vi "Set_Adam_Watchdogs.vi"(1 "Set Watchdogs":bool) -> (0 "Error String":string)   [LabVIEW 2016]
uses:
  Anemometry/Anemometry Sub Vis/Globals/Constants_global.vi
panel:
  out "Day Time":bool
  out "Display":string[][](table)
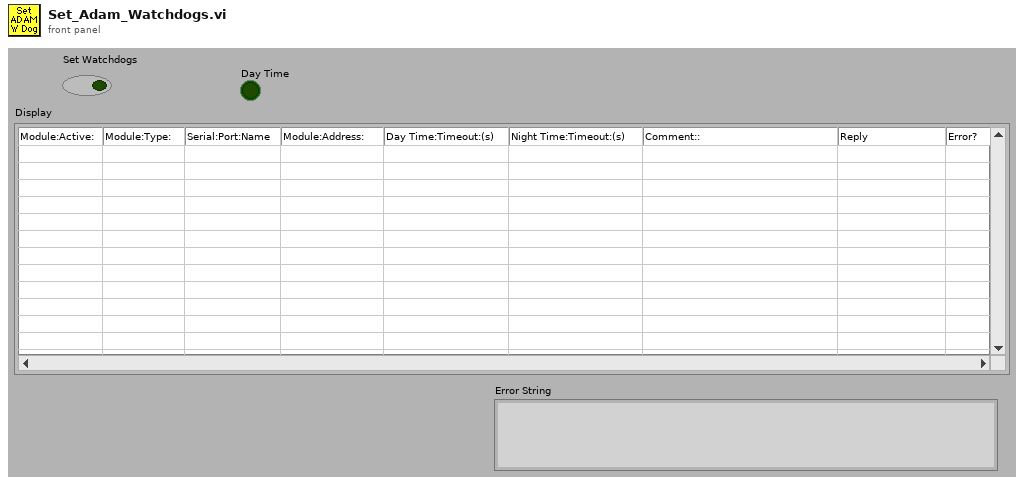
[diagram p1: front panel]
types:
  T1 = typedef "LVDateTimeRec.ctl" = cluster{"fractional second":dbl, "second":i32, "minute":i32, "hour":i32, "day of month":i32, "month":i32, "year":i32, "day of week":i32, "day of year":i32, "DST":i32}
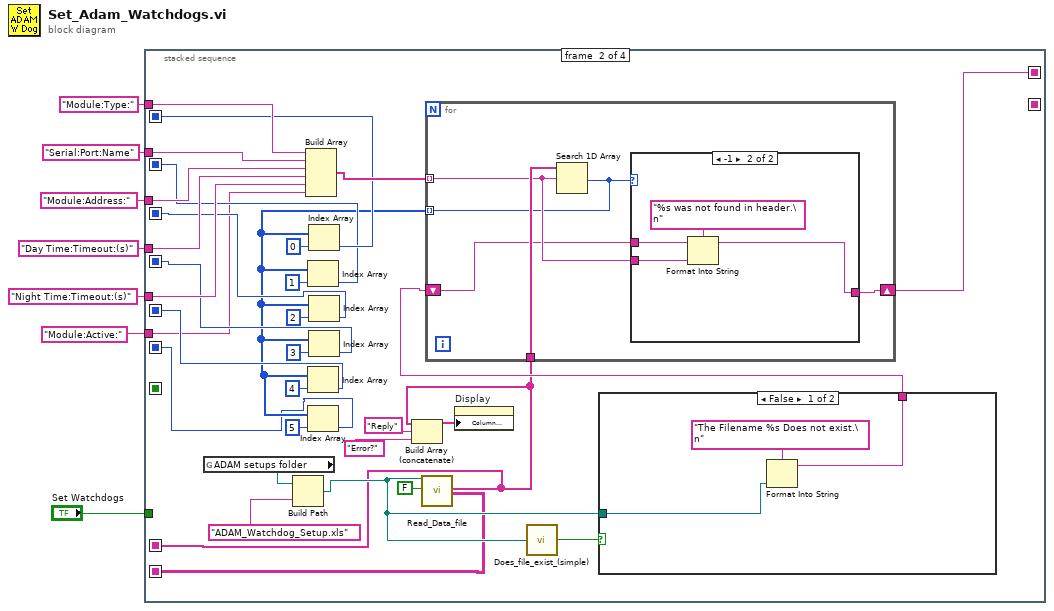
[diagram p0: block diagram]
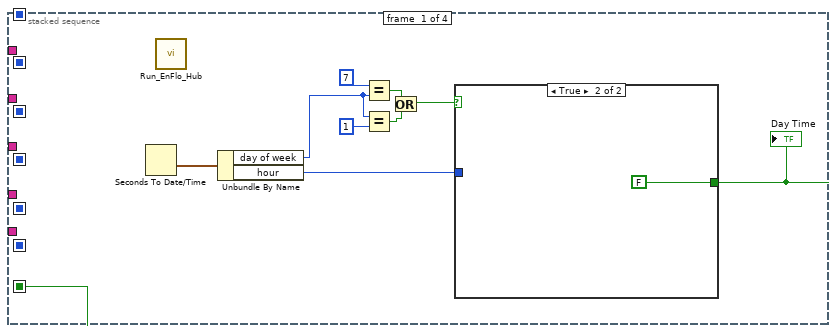
[diagram p2: hidden frame]
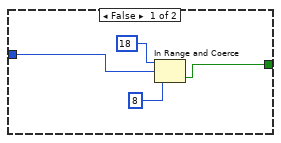
[diagram p3: hidden frame]
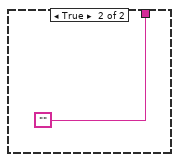
[diagram p4: hidden frame]
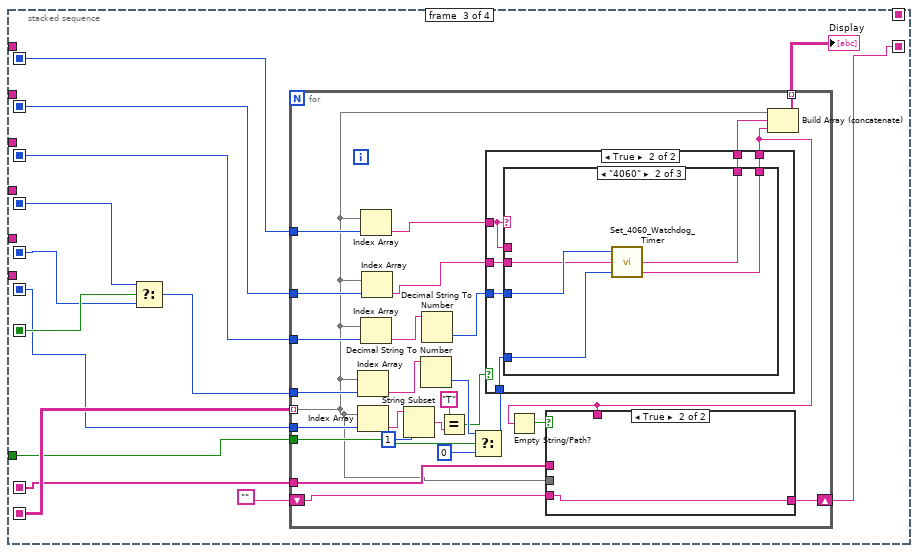
[diagram p6: hidden frame]
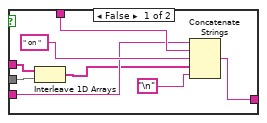
[diagram p7: hidden frame]
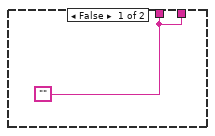
[diagram p8: hidden frame]
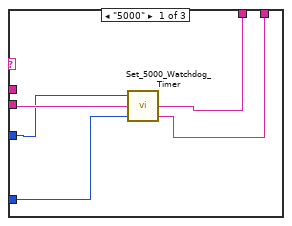
[diagram p9: hidden frame]
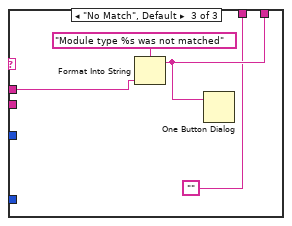
[diagram p10: hidden frame]
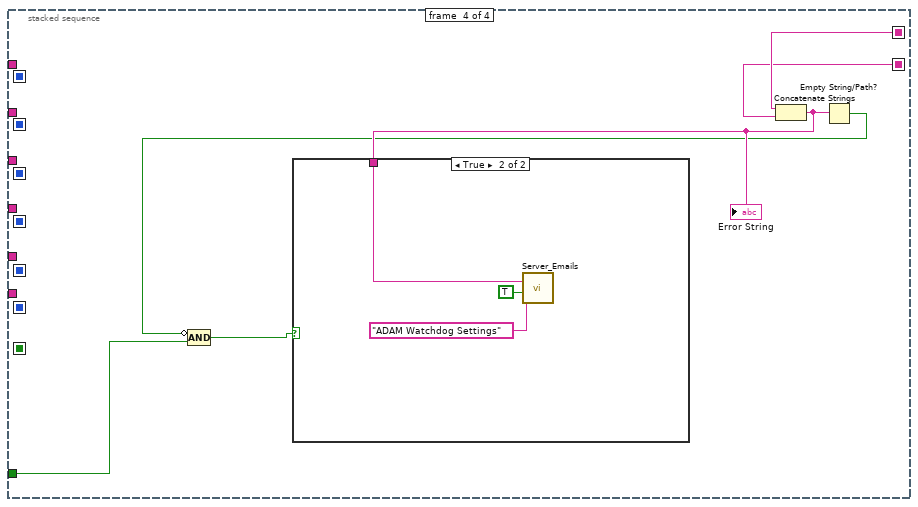
[diagram p11: hidden frame]
diagram:
  n1 = stacked-sequence {
    seq-local: [w8 _ _ _] -> [_ _ w80 _]
    seq-local: [_ w36 _ _] -> [_ _ w78 _]
    seq-local: [_ w35 _ _] -> [_ _ w77 _]
    seq-local: [_ w34 _ _] -> [_ _ w76 _]
    seq-local: [_ w33 _ _] -> [_ _ w75 _]
    seq-local: [_ w32 _ _] -> [_ _ w74 _]
    seq-local: [_ w42 _ _] -> [_ _ _ w144]
    seq-local: [_ w31 _ _] -> [_ _ w79 _]
    seq-local: [_ _ w71 _] -> [_ _ _ w143]
    seq-local: [_ w24 _ _] -> [_ _ w69 _]
    seq-local: [_ w23 _ _] -> [_ _ w68 _]
    tunnel: "Module:Type:" -> [_ w51 _ _]
    tunnel: "Serial:Port:Name" -> [_ w50 _ _]
    tunnel: "Module:Address:" -> [_ w49 _ _]
    tunnel: "Day Time:Timeout:(s)" -> [_ w48 _ _]
    tunnel: "Night Time:Timeout:(s)" -> [_ w47 _ _]
    tunnel: "Set Watchdogs" -> [_ _ w70 w141]
    tunnel: "Module:Active:" -> [_ w27 _ _]
    frame #0 {
      n2 = Seconds To Date/Time() -> (date time rec=w9:T1)  [unwired: 2 in]
      n3 = call "Run_EnFlo_Hub.vi"() -> ()  [unwired: 7 in, 1 out]
      n4 = Unbundle By Name(w9) -> ("day of week"=w11:i32, "hour"=w16:i32)
      n5 = Equal?(x=7, y=w11) -> (x = y?=w13:bool)
      n6 = Equal?(x=w11, y=1) -> (x = y?=w14:bool)
      n7 = Or(x=w13, y=w14) -> (x .or. y?=w15:bool)
      n8 = case shown="True" w15 {
        tunnel: w16 -> [w20 _]
        tunnel: [w17 FALSE] -> w8
        frame False {
          n9 = In Range and Coerce(upper limit=18, x=w20, lower limit=8) -> (In Range?=w17:bool)  [unwired: 1 out]
        }
        frame True {
        }
      }
      "Day Time" <- w8
    }
    frame #1 {
      n10 = global read "Constants_global.vi" "ADAM setups folder"() -> (w53:path)
      n11 = Build Path(base path=w53, name or relative path="ADAM_Watchdog_Setup.xls") -> (appended path=w44:path)
      n12 = Build Array(w51, w50, w49, w48, w47, w27) -> (w46:string[])
      n13 = call "Read_Data_file.vi"("Results file"=w44, "Delete First Rows?"=FALSE) -> ("Ch names Out"=w23:string[], "Channel Values Out"=w31:string[][])  [unwired: 7 in, 9 out]
      n14 = Build Array (concatenate)(w23, "Reply", "Error?" ("element")) -> (w29:string[])
      n15 = property on="Display" class="Tbl (strict)"("Column Headers[]"=w29) -> ()  [unwired: 2 in, 2 out]
      n16 = call "Does_file_exist_(simple).vi"("Pathname"=w44) -> ("exists?"=w45:bool)
      n17 = case shown="False" w45 {
        tunnel: w44 -> [w56 _]
        tunnel: [w54 ""] -> w43
        frame False {
          n18 = Format Into String(format string="The Filename %s Does not exist.\n", w56) -> (resulting string=w54:string)  [unwired: 2 in, 1 out]
        }
        frame True {
        }
      }
      n19 = for {
        tunnel: w23 -> [w62]
        tunnel: w46 -> [w61] mode=indexing
        shift-right: [w59] -> w42
        shift-left: w43 -> [w60]
        tunnel: [w58] -> w25 mode=indexing
        n20 = Search 1D Array(1D array=w62, element=w61) -> (index of element=w58:i32)  [unwired: 1 in]
        n21 = case shown="-1" w58 {
          tunnel: w61 -> [_ w67]
          tunnel: w60 -> [w63 w65]
          tunnel: [w63 w64] -> w59
          frame 0, Default {
          }
          frame -1 {
            n22 = Format Into String(format string="%s was not found in header.\n", initial string=w65, w67) -> (resulting string=w64:string)  [unwired: 1 in, 1 out]
          }
        }
      }
      n23 = Index Array(array=w25, index=1) -> (element=w35:i32)
      n24 = Index Array(array=w25, index=4) -> (element=w32:i32)
      n25 = Index Array(array=w25, index=5) -> (element=w24:i32)
      n26 = Index Array(array=w25, index=0) -> (element=w36:i32)
      n27 = Index Array(array=w25, index=2) -> (element=w34:i32)
      n28 = Index Array(array=w25, index=3) -> (element=w33:i32)
    }
    frame #2 {
      n29 = Select(t=w75, s=w80, f=w74) -> (s? t:f=w73:i32)
      n30 = for {
        tunnel: w79 -> [w85] mode=indexing
        tunnel: w70 -> [w103]
        tunnel: [w98] -> w81 mode=indexing
        tunnel: w78 -> [w97]
        tunnel: w77 -> [w96]
        tunnel: w76 -> [w95]
        tunnel: w73 -> [w94]
        shift-right: [w82] -> w71
        shift-left: "" -> [w83]
        tunnel: w69 -> [w93]
        tunnel: w68 -> [w86]
        n31 = Index Array(array=w85, index=w94) -> (element=w104:string)
        n32 = Index Array(array=w85, index=w93) -> (element=w91:string)
        n33 = Index Array(array=w85, index=w97) -> (element=w108:string)
        n34 = Index Array(array=w85, index=w95) -> (element=w106:string)
        n35 = Index Array(array=w85, index=w96) -> (element=w105:string)
        n36 = String Subset(string=w91, length (rest)=1 ("length (rest)")) -> (substring=w90:string)  [unwired: 1 in]
        n37 = Decimal String To Number(string=w104) -> (number=w102:i32)  [unwired: 2 in, 1 out]
        n38 = Decimal String To Number(string=w106) -> (number=w107:i32)  [unwired: 2 in, 1 out]
        n39 = Equal?(x="T", y=w90) -> (x = y?=w88:bool)
        n40 = Select(t=w102, s=w103, f=0) -> (s? t:f=w100:i32)
        n41 = case shown="True" w88 {
          tunnel: w108 -> [_ w119]
          tunnel: w107 -> [_ w124]
          tunnel: w105 -> [_ w123]
          tunnel: w100 -> [_ w122]
          tunnel: [w118 w121] -> w99
          tunnel: [w118 w120] -> w84
          frame False {
            w118 = ""
          }
          frame True {
            n42 = case shown="\"4060\"" w119 {
              tunnel: w119 -> [_ _ w138]
              tunnel: w124 -> [w128 w134 _]
              tunnel: w123 -> [w129 w133 _]
              tunnel: w122 -> [w127 w132 _]
              tunnel: [w126 w131 ""] -> w121
              tunnel: [w125 w130 w136] -> w120
              frame "5000" {
                n43 = call "Set_5000_Watchdog_Timer.vi"("Watchdog Timer  Seconds"=w127, "Port Name"=w129, "Module Address"=w128) -> ("Comment out"=w125:string, "Reply"=w126:string)  [unwired: 1 out]
              }
              frame "4060" {
                n44 = call "Set_4060_Watchdog_Timer.vi"("Watchdog Timer  Seconds"=w132, "Port Name"=w133, "Module Address"=w134) -> ("Comment out"=w130:string, "Reply"=w131:string)  [unwired: 1 out]
              }
              frame "No Match", Default {
                n45 = Format Into String(format string="Module type %s was not matched", w138) -> (resulting string=w136:string)  [unwired: 2 in, 1 out]
                n46 = One Button Dialog(message=w136) -> ()  [unwired: 1 in, 1 out]
              }
            }
          }
        }
        n47 = Empty String/Path?(string/path=w84) -> (empty?=w87:bool)
        n48 = case shown="True" w87 {
          tunnel: w86 -> [w113 _]
          tunnel: w85 -> [w116 _]
          tunnel: w84 -> [w115 _]
          tunnel: w83 -> [w111 w117]
          tunnel: [w112 w117] -> w82
          frame False {
            n49 = Interleave 1D Arrays(w113, w116) -> (w110:string[])
            n50 = Concatenate Strings(w111, w115, " on ", w110, "\n") -> (w112:string)
          }
          frame True {
          }
        }
        n51 = Build Array (concatenate)(w85, w99, w84) -> (w98:string[])
      }
      "Display" <- w81
    }
    frame #3 {
      n52 = Concatenate Strings(w144, w143) -> (w142:string)
      "Error String" <- w142
      n53 = Empty String/Path?(string/path=w142) -> (empty?=w140:bool)
      n54 = Compound Arithmetic op=AND(invert w140, w141) -> (w139:bool)
      n55 = case shown="True" w139 {
        tunnel: w142 -> [_ w145]
        frame False {
        }
        frame True {
          n56 = call "Server_Emails.vi"("Message"=w145, "Contact All clients?"=TRUE, "Subject"="ADAM Watchdog Settings") -> ()  [unwired: 2 in, 3 out]
        }
      }
    }
  }
